vi "Wind_Turbine_Control.vi"(3 "Mode":T5=enum."Run VI", 5 "Traverse line In":T2={"Start X"=0.0, "Start Y"=0.0, "Start Z"=0.0, "End X"=0.0, "End Y"=0.0, "End Z"=0.0, "nPoints"=0, "Spacing"=enum."Linear", "Filename"=path "", "Tunnel Speed"=0.0, "Averaging time (mins)"=0.0, "Extra Commands"="0.02 ; 1.0", "Carrier_1 Q (l/min)"=0.0, "Carrier_2 Q (l/min)"=0.0, "Trace Gas Concentration (%)"=0.0, "Specific Arguments"="Wind_Turbine_Control.vi; 600", "Comments"="", "Row No"=0, "Row Type Selector"=enum."Move Traverse Only", "EstCompl"="", "Row Duration (mins)"=0.0, "nValidPoints"=0, "Meas Setup File"=""} {"Carrier_2 Q (l/min)" format="%#.2f"; "Row Duration (mins)" format="%#.1f"; "Row No" min=0; "Trace Gas Concentration (%)" min=0.0 format="%#_4f"; "Carrier_1 Q (l/min)" format="%#.4f"; "Start X" format="%#.2f"; "Start Y" format="%#.2f"; "Start Z" format="%#.2f"; "End X" format="%#.2f"; "End Y" format="%#.2f"; "End Z" format="%#.2f"; "Tunnel Speed" format="%#.2f"; "Averaging time (mins)" min=0.0 format="%#.2f"}) -> (0 "Error Message":string, 1 "Status":T1, 2 "Traverse line Out":T2={"Start X"=0.0, "Start Y"=0.0, "Start Z"=0.0, "End X"=0.0, "End Y"=0.0, "End Z"=0.0, "nPoints"=0, "Spacing"=enum."Linear", "Filename"=path "", "Tunnel Speed"=0.0, "Averaging time (mins)"=0.0, "Extra Commands"="0.035 ; 0.1", "Carrier_1 Q (l/min)"=0.0, "Carrier_2 Q (l/min)"=0.0, "Trace Gas Concentration (%)"=0.0, "Specific Arguments"="Wind_Turbine_Control.vi; 600", "Comments"="", "Row No"=0, "Row Type Selector"=enum."Move Traverse Only", "EstCompl"="", "Row Duration (mins)"=0.0, "nValidPoints"=0, "Meas Setup File"=""} {"Carrier_2 Q (l/min)" format="%#.2f"; "Row Duration (mins)" format="%#.1f"; "Row No" min=0; "Trace Gas Concentration (%)" min=0.0 format="%#_4f"; "Carrier_1 Q (l/min)" format="%#.4f"; "Start X" format="%#.2f"; "Start Y" format="%#.2f"; "Start Z" format="%#.2f"; "End X" format="%#.2f"; "End Y" format="%#.2f"; "End Z" format="%#.2f"; "Tunnel Speed" format="%#.2f"; "Averaging time (mins)" min=0.0 format="%#.2f"})   [LabVIEW 2021]
uses:
  Gen Trav/Traverse_cluster.ctl
  Gen Trav/Spacing.ctl
  Controls/Multi_run_mode.ctl
  Controls/User_Specific_mode.ctl
  Gen Trav/Multi_Run_Status.ctl
panel:
  in  "RS-485 addr.":u8
  # "X           Y          Z"
  # "Start"
  # "End"
  # "X           Y          Z"
  # "Start"
  # "End"
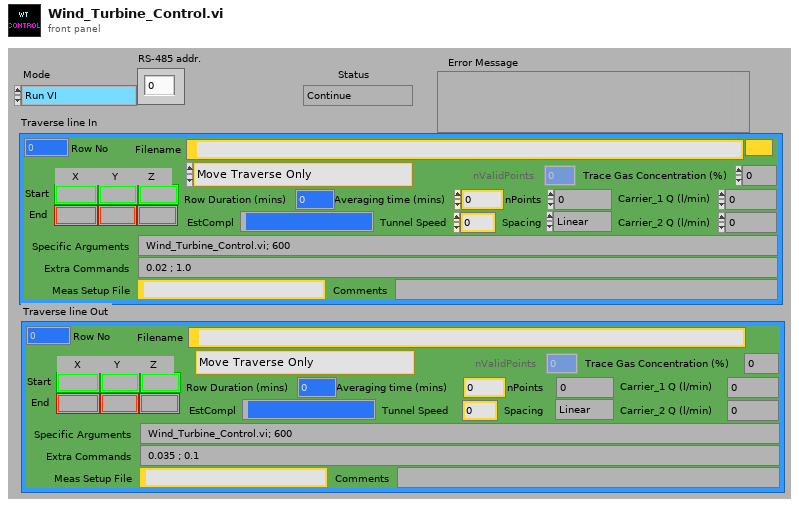
[diagram p1: front panel]
types:
  T1 = typedef "Multi_Run_Status.ctl" = enum16{"Continue", "Continue with Error", "Jump to Next Point", "Jump to Next Row", "Jump To Fall Back", "Terminate Run"}
  T2 = typedef "Traverse_cluster.ctl" = cluster{"Start X":sgl, "Start Y":sgl, "Start Z":sgl, "End X":sgl, "End Y":sgl, "End Z":sgl, "nPoints":i32, "Spacing":T3, "Filename":path, "Tunnel Speed":dbl, "Averaging time (mins)":dbl, "Extra Commands":string, "Carrier_1 Q (l/min)":dbl, "Carrier_2 Q (l/min)":dbl, "Trace Gas Concentration (%)":dbl, "Specific Arguments":string, "Comments":string, "Row No":i32, "Row Type Selector":T4, "EstCompl":string, "Row Duration (mins)":dbl, "nValidPoints":i32, "Meas Setup File":string}
  T3 = typedef "Spacing.ctl" = enum16{"Linear", "Log", "Gauss", "Specified", "N/A"}
  T4 = typedef "Multi_run_mode.ctl" = enum16{"Move Traverse Only", "Set Tunnel Speed Only", "Set Source Only", "Set Measurement Conditions", "Single Measurement", "Vertical Profile", "Lateral Profile", "Longitudinal Profile", "Multi-Axis Profile", "Explore Volume", "Auto Calibrate", "Meas Fast FID Bkgnd", "Check Beam Power", "Scanning Valve Measurement", "Run VI Named:", "Set ADAM Ch", "Wait (minutes)", "Send Message", "Synchronize With:", "Fall Back to this Row", "Turn Off Row Repeating", "Traverse 3D Volume", "Blank Row", "Jump to Fall Back Row"}
  T5 = typedef "User_Specific_mode.ctl" = enum16{"Check VI only", "Run VI"}
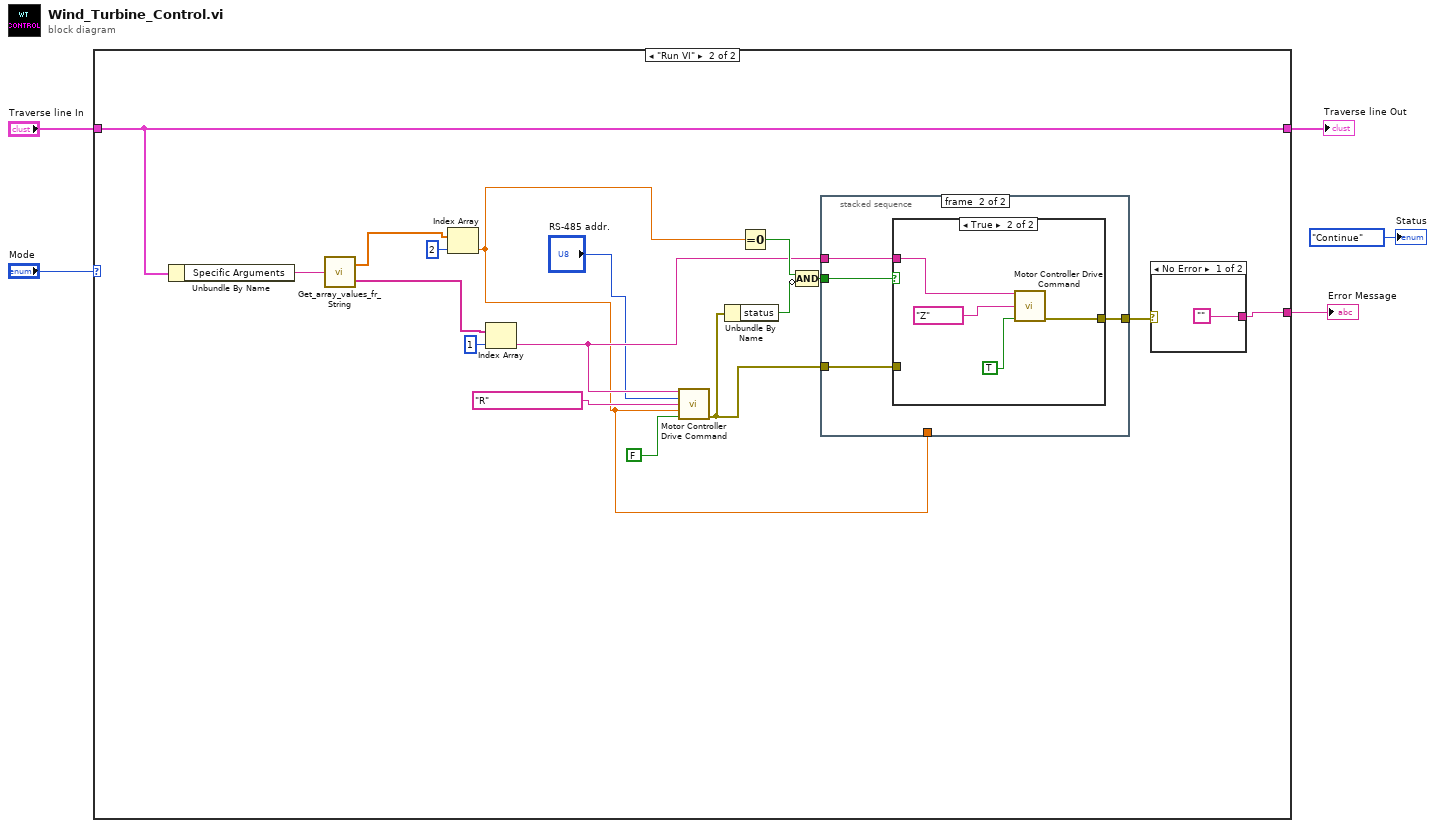
[diagram p0: block diagram]
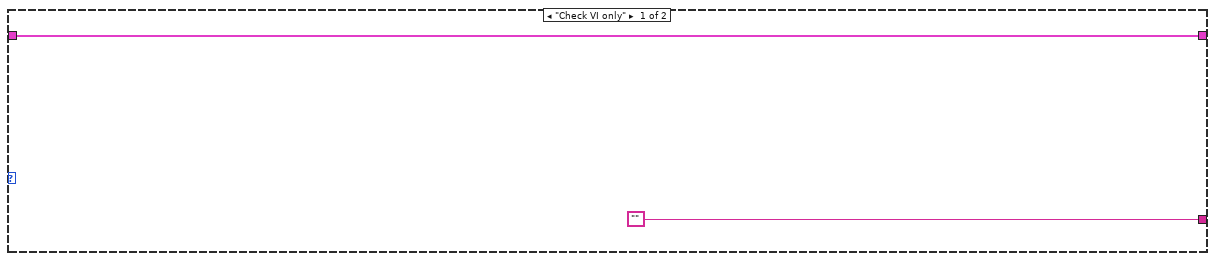
[diagram p2: hidden frame]
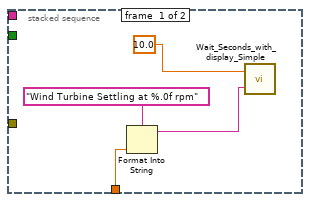
[diagram p3: hidden frame]
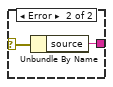
[diagram p5: hidden frame]
diagram:
  n1 = case shown="\"Run VI\"" "Mode" {
    tunnel: "Traverse line In" -> [w7 w24]
    tunnel: [w7 w24] -> w3
    tunnel: ["" w22] -> w2
    frame "Check VI only" {
    }
    frame "Run VI" {
      n2 = Unbundle By Name(w24) -> ("Specific Arguments"=w23:string)
      n3 = call "Get_array_values_fr_String.vi"("String Value"=w23) -> ("Numeric Array"=w21:dbl[], "String array"=w20:string[])
      n4 = Index Array(array=w21, index=2) -> (element=w8:dbl)
      n5 = Index Array(array=w20, index=1) -> (element=w13:string)
      n6 = call "Motor Controller Drive Command.vi"("COM port"=w13, "RS-485 addr."="RS-485 addr.", "Command"="R", "RPM setpoint"=w8, "Close port after action"=FALSE) -> ("Error out"=w9:errorcluster)  [unwired: 9 in, 1 out]
      n7 = Unbundle By Name(w9) -> ("status"=w17:bool)
      n8 = Equal To 0?(x=w8) -> (x = 0?=w16:bool)
      n9 = Compound Arithmetic op=AND(w16, invert w17) -> (w15:bool)
      n10 = stacked-sequence {
        tunnel: w15 -> [_ w32]
        tunnel: [_ w31] -> w14
        tunnel: w13 -> [_ w30]
        tunnel: w9 -> [_ w29]
        tunnel: w8 -> [w27 _]
        frame #0 {
          n11 = Format Into String(format string="Wind Turbine Settling at %.0f rpm", w27) -> (resulting string=w25:string)  [unwired: 2 in, 1 out]
          n12 = call "Wait_Seconds_with_display_Simple.vi"("Message"=w25, "Seconds to wait"=10.0) -> ()  [unwired: 1 in, 1 out]
        }
        frame #1 {
          n13 = case shown="True" w32 {
            tunnel: w30 -> [_ w37]
            tunnel: [w33 w35] -> w31
            tunnel: w29 -> [w33 _]
            frame False {
            }
            frame True {
              n14 = call "Motor Controller Drive Command.vi"("COM port"=w37, "Command"="Z", "Close port after action"=TRUE) -> ("Error out"=w35:errorcluster)  [unwired: 11 in, 1 out]
            }
          }
        }
      }
      n15 = case shown="No Error" w14 {
        selector: w14 -> [_ w39]
        tunnel: ["" w40] -> w22
        frame No Error {
        }
        frame Error {
          n16 = Unbundle By Name(w39) -> ("source"=w40:string)
        }
      }
    }
  }
  "Traverse line Out" <- w3
  "Error Message" <- w2
  "Status" <- Multi_Run_Status."Continue" ("Status")
